vi "server.Send Request (Batch Async).vi"(8 "error in (no error)":errorcluster, 10 "JSON Request String":string[](array[string]), 11 "Server in":refnum<class "JSONRPC Server.lvclass">) -> (0 "error out":errorcluster, 1 "notification?":bool[](array[boolean]), 2 "id value":string[](array[string]), 3 "Server out":refnum<class "JSONRPC Server.lvclass">)   [LabVIEW 2016, in "JSONRPC Server.lvclass"]
uses:
  JSONRPC Server.lvclass
  Request/Request.lvclass
  Request/Request.lvclass/Request.ctl
  Request/request.Has ID.vi
  Request/request.Read id value.vi
  id/id.Read value.vi
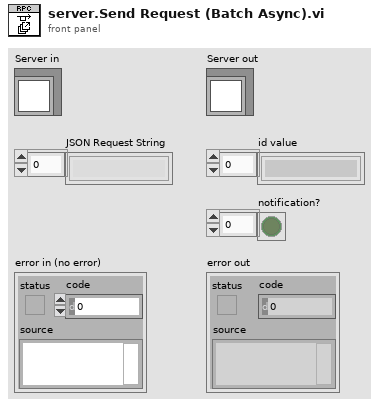
[diagram p1: front panel]
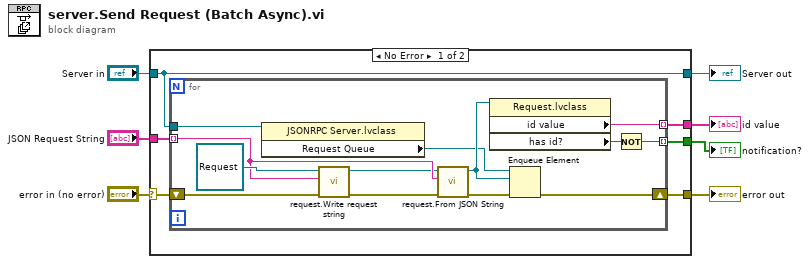
[diagram p0: block diagram]
diagram:
  n1 = case shown="No Error" "error in (no error)" {
    selector: "error in (no error)" -> [w8 w28]
    tunnel: [w12 w28] -> w4
    tunnel: [w13 w27] -> w3
    tunnel: "Server in" -> [w13 w27]
    tunnel: "JSON Request String" -> [w9 _]
    tunnel: [w11 _] -> w2
    tunnel: [w10 _] -> w1
    frame No Error {
      n2 = for {
        tunnel: w13 -> [w16]
        tunnel: [w23] -> w11 mode=indexing
        tunnel: [w21] -> w10 mode=indexing
        tunnel: w9 -> [w19] mode=indexing
        shift-right: [w25] -> w12
        shift-left: w8 -> [w18]
        n3 = property class="JSONRPC Server.lvclass"(reference=w16) -> ("Request Queue"=w15:refnum<queue>)  [unwired: 1 in, 2 out]
        n4 = call "request.Write request string.vi"("error in (no error)"=w18, "request string"=w19, "Request in"=refnum<class "Request.lvclass"> refnum ("Request.lvclass")) -> ("error out"=w17:errorcluster, "Request out"=w14:refnum<class "Request.lvclass">)  [unwired: 7 in]
        n5 = call "request.From JSON String.vi"("error in (no error)"=w17, "JSON String"=w19, "Request in"=w14) -> ("error out"=w26:errorcluster, "Request out"=w24:refnum<class "Request.lvclass">)  [unwired: 7 in]
        n6 = property class="Request.lvclass"(reference=w24) -> ("id value"=w23:string, "has id?"=w22:bool)  [unwired: 1 in, 2 out]
        n7 = Enqueue Element(queue=w15, element=w24, error in (no error)=w26) -> (error out=w25:errorcluster)  [unwired: 1 in, 2 out]
        n8 = Not(x=w22) -> (.not. x?=w21:bool)
      }
    }
    frame Error {
    }
  }
  "error out" <- w4
  "Server out" <- w3
  "id value" <- w2
  "notification?" <- w1
